vi "formatIntoHighlightedRows.vi"(8 "error in (no error)":errorcluster, 11 "OutcomeList in":refnum<class "OutcomeList.lvclass">) -> (0 "error out":errorcluster, 2 "Highlighted Rows":i32[](array[numeric]), 3 "OutcomeList out":refnum<class "OutcomeList.lvclass">)   [LabVIEW 2018, in "OutcomeList.lvclass"]
uses:
  OutcomeList.lvclass
  OutcomeList.lvclass/OutcomeList.ctl
  Expense Summary/Outcome.lvclass
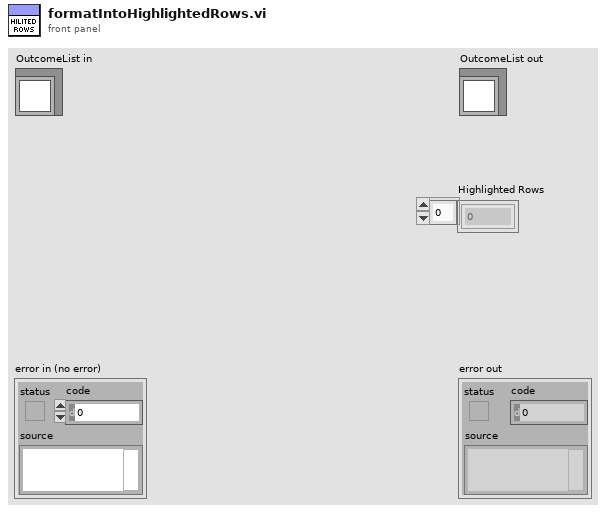
[diagram p1: front panel]
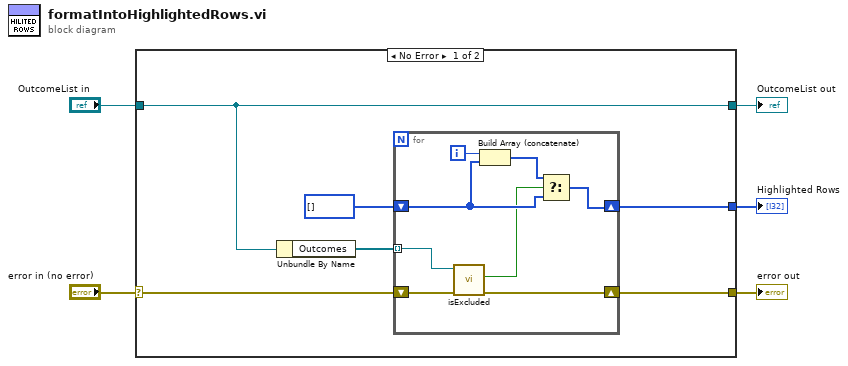
[diagram p0: block diagram]
diagram:
  n1 = case shown="No Error" "error in (no error)" {
    selector: "error in (no error)" -> [w8 w21]
    tunnel: [w7 w21] -> w4
    tunnel: [w9 w20] -> w2
    tunnel: "OutcomeList in" -> [w9 w20]
    tunnel: [w6 _] -> w1
    frame No Error {
      n2 = Unbundle By Name(w9) -> ("Outcomes"=w11:refnum<class "Outcome.lvclass">[])
      n3 = for {
        tunnel: w11 -> [w12] mode=indexing
        shift-right: [w14] -> w7
        shift-left: w8 -> [w15]
        shift-right: [w19] -> w6
        shift-left: i32[] [] ("Highlighted Rows") -> [w17]
        i -> [w18]
        n4 = call "isExcluded.vi"("error in (no error)"=w15, "Outcome in"=w12) -> ("error out"=w14:errorcluster, "Excluded?"=w13:bool)  [unwired: 7 in, 1 out]
        n5 = Build Array (concatenate)(w18, w17) -> (w16:i32[])
        n6 = Select(t=w16, s=w13, f=w17) -> (s? t:f=w19:i32[])
      }
    }
    frame Error {
    }
  }
  "error out" <- w4
  "OutcomeList out" <- w2
  "Highlighted Rows" <- w1
